vi "Init SPI.vi"(5 "SPI Config":T1={"Mode"=0, "Data Bits"=8, "MOSI Pin"=0, "MISO Pin"=0, "SCK Pin"=0}, 7 "Bus":u8, 8 "error in (no error)":errorcluster, 10 "Baud":u32 format="%.0p", 11 "VISA resource name in":refnum<visa-resource-name>) -> (0 "error out":errorcluster, 3 "VISA resource name":refnum<visa-resource-name>)   [LabVIEW 2023, in "CTI-Visa.lvlib"]
uses:
  CTI-Visa.lvlib
  SPI Config.ctl
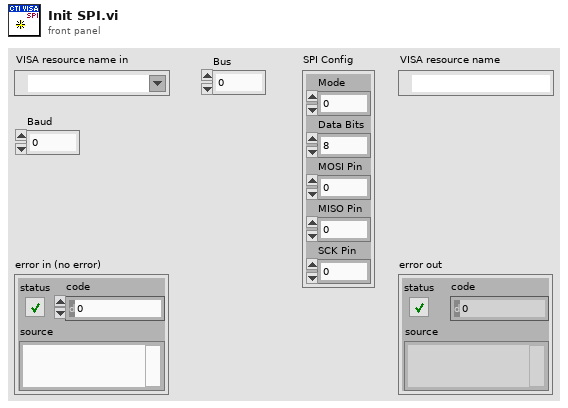
[diagram p1: front panel]
types:
  T1 = typedef "CTI-Visa.lvlib/SPI Config.ctl" = cluster{"Mode":u8, "Data Bits":u8, "MOSI Pin":u8, "MISO Pin":u8, "SCK Pin":u8}
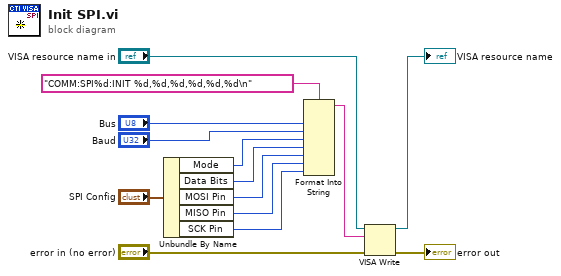
[diagram p0: block diagram]
diagram:
  n1 = Unbundle By Name("SPI Config") -> ("Mode"=w5:u8, "Data Bits"=w4:u8, "MOSI Pin"=w3:u8, "MISO Pin"=w2:u8, "SCK Pin"=w1:u8)
  n2 = Format Into String(format string="COMM:SPI%d:INIT %d,%d,%d,%d,%d,%d\n", "Bus", "Baud", w5, w4, w3, w2, w1) -> (resulting string=w9:string)  [unwired: 2 in, 1 out]
  n3 = VISA Write(VISA resource name="VISA resource name in", write buffer=w9, error in (no error)="error in (no error)") -> (VISA resource name out=→"VISA resource name":refnum<visa-resource-name>, error out=→"error out":errorcluster)  [unwired: 1 out]
